vi "Send Close Message.vi"(8 "error in (no error)":errorcluster, 11 "MessageQ":refnum<class "MessageQ.lvclass">) -> (0 "error out":errorcluster)   [LabVIEW 2020, in "Volatus.lvlib"]
uses:
  Volatus.lvlib
  MessageQ/MessageQ.lvclass
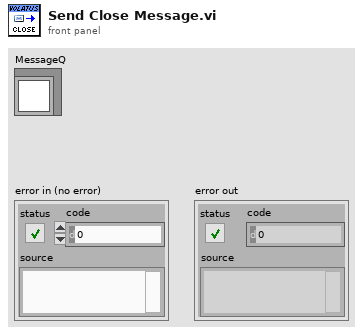
[diagram p1: front panel]
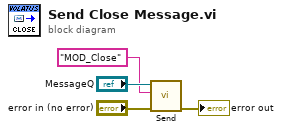
[diagram p0: block diagram]
diagram:
  n1 = call "Send.vi"("error in (no error)"="error in (no error)", "ID"="MOD_Close", "MessageQ in"="MessageQ") -> ("error out"=→"error out":errorcluster)  [unwired: 7 in, 1 out]
